vi "ESP_Q_vel.vi"(8 "error in (no error)":errorcluster, 9 "Position":dbl, 10 "Axis":T1(ring), 11 "queue":refnum<queue>) -> (0 "error out":errorcluster, 3 "queue out":refnum<queue>)   [LabVIEW 2020]
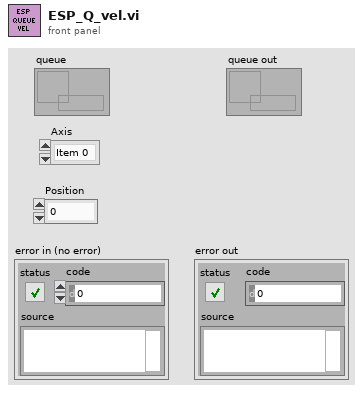
[diagram p1: front panel]
types:
  T1 = enum32{"Item 0", "Item 1", "Radio Selection 3", "Radio Selection 4", "Radio Selection 5"}
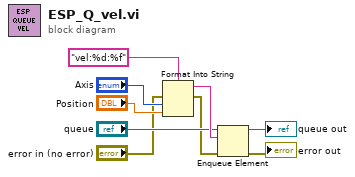
[diagram p0: block diagram]
diagram:
  n1 = Format Into String(format string="vel:%d:%f", error in="error in (no error)", "Axis", "Position") -> (resulting string=w9:string, error out=w2:errorcluster)  [unwired: 1 in]
  n2 = Enqueue Element(queue="queue", element=w9, error in (no error)=w2) -> (queue out=→"queue out":refnum<queue>, error out=→"error out":errorcluster)  [unwired: 1 in, 1 out]
